vi "Write Section Path.vi"(7 "Section Name":string, 8 "error in (no error)":errorcluster, 9 "create file if necessary (T)":bool=TRUE, 10 "Section (Cluster)":variant, 11 "Path in":path) -> (0 "error out":errorcluster, 1 "file created?":bool, 3 "Path out":path)   [LabVIEW 2020, in "Generic Config Handling.lvlib"]
doc: "This vi writes the cluster as a section in the config file. \n\nIf section name is not wired then the default is to use the name of the cluster.\n\nEach element of the cluster becomes a key, therefore it must be named, and they should be unique and not include any special characters (spaces are allowed and are replaced by_)\n\nYou cannot nest clusters and only simple datatypes are allowed. 1D and 2D arrays are allowed. They are stored as a single element with columns delimited by semicolons and rows delimited by commas. 1D arrays are stored as a single row (ie. comma delimited). \n\nEnums are stored as U32s."
uses:
  Generic Config Handling.lvlib
  <vilib>/Utility/config.llb/NI_LVConfig.lvlib
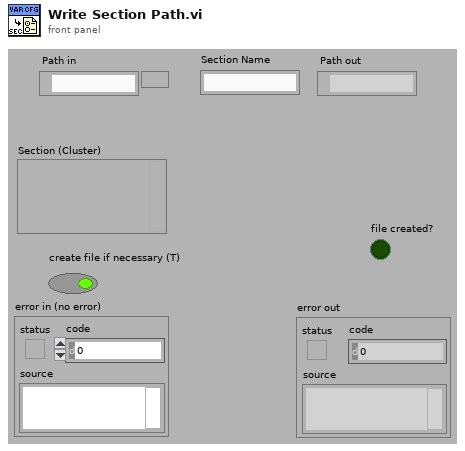
[diagram p1: front panel]
types:
  T1 = typedef "NI_LVConfig.lvlib/Config Data RefNum.ctl" = refnum<k1>
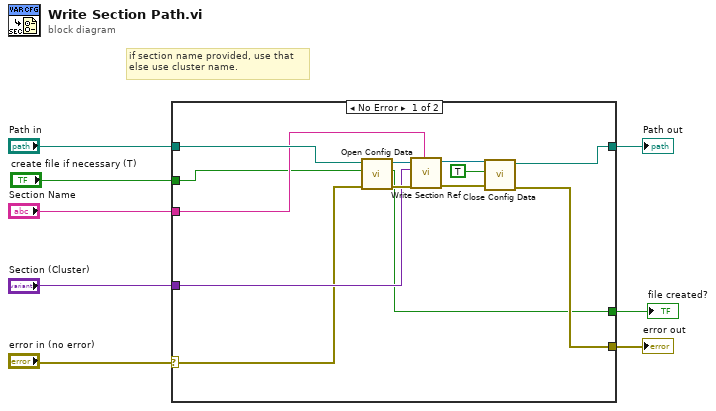
[diagram p0: block diagram]
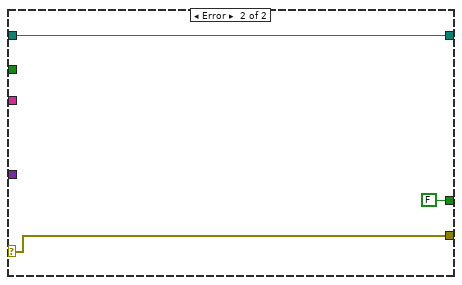
[diagram p2: hidden frame]
diagram:
  # "if section name provided, use that\nelse use cluster name."
  n1 = case shown="No Error" "error in (no error)" {
    selector: "error in (no error)" -> [w9 w23]
    tunnel: "Path in" -> [w19 w24]
    tunnel: "Section (Cluster)" -> [w18 _]
    tunnel: [w14 w24] -> w6
    tunnel: [w13 w23] -> w5
    tunnel: "Section Name" -> [w12 _]
    tunnel: "create file if necessary (T)" -> [w11 _]
    tunnel: [w10 FALSE ("file created?")] -> w2
    frame No Error {
      n2 = call <vilib>:"Open Config Data.vi"("error in (no error)"=w9, "create file if necessary (T)"=w11, "configuration file path"=w19) -> ("error out"=w20:errorcluster, "file created?"=w10:bool, "refnum"=w21:T1)  [unwired: 6 in]
      n3 = call "Write Section Ref.vi"("Section Name"=w12, "error in (no error)"=w20, "Section (Cluster)"=w18, "Refnum in"=w21) -> ("error out"=w16:errorcluster, "Refnum out"=w17:T1)  [unwired: 6 in]
      n4 = call <vilib>:"Close Config Data.vi"("error in (no error)"=w16, "write file if changed (T)"=TRUE, "refnum"=w17) -> ("error out"=w13:errorcluster, "file path"=w14:path)  [unwired: 7 in]
    }
    frame Error {
    }
  }
  "Path out" <- w6
  "error out" <- w5
  "file created?" <- w2
